vi "BinF_ReadData.vi"(6 "Channel number":i64, 7 "BinF File Settings":T1={"Version"=2, "Data Representation"=enum."I16", "# columns (samples per channel)"=300, "# rows (channels)"=150, "# pre-trigger samples"=20, "Sample rate"=1000.0, "ADC offset"=256.0, "Scale factor"=0.001}, 8 "error in":errorcluster, 9 "Length":i32, 10 "Start":i64, 11 "refnum":refnum<file>) -> (0 "error out":errorcluster, 1 "Unscaled data":sgl[](array[numeric]), 2 "Channel Data":sgl[](array[numeric]), 3 "refnum out":refnum<file>)   [LabVIEW 2021]
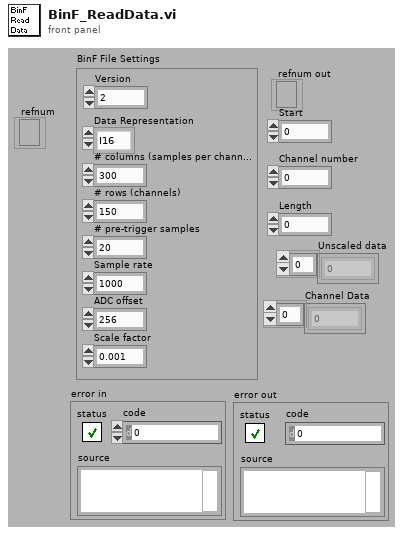
[diagram p1: front panel]
types:
  T1 = cluster{"Version":i16, "Data Representation":enum16{"Undefined", "I8", "I16", "I32", "I64", "U8", "U16", "U32", "U64", "SGL", "DBL", "EXT"}, "# columns (samples per channel)":i64, "# rows (channels)":i64, "# pre-trigger samples":i64, "Sample rate":dbl, "ADC offset":dbl, "Scale factor":dbl}
  T2 = enum16{"Undefined", "I8", "I16", "I32", "I64", "U8", "U16", "U32", "U64", "SGL", "DBL", "EXT"}
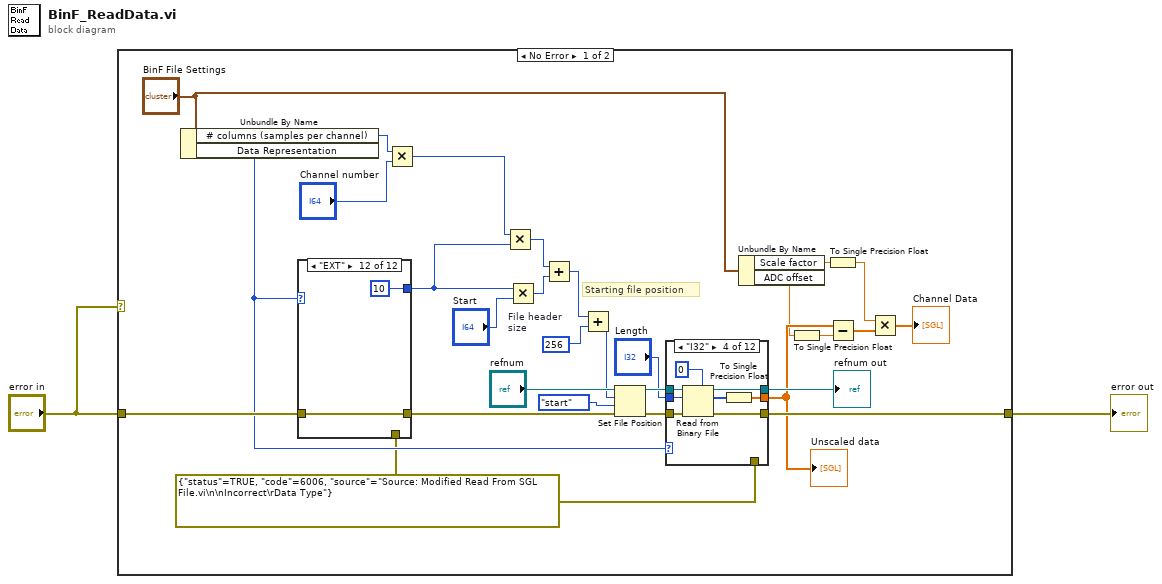
[diagram p0: block diagram]
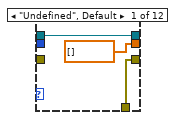
[diagram p2: hidden frame]
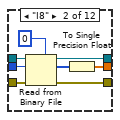
[diagram p3: hidden frame]
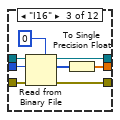
[diagram p4: hidden frame]
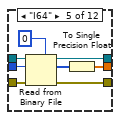
[diagram p5: hidden frame]
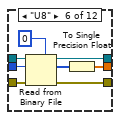
[diagram p6: hidden frame]
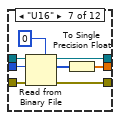
[diagram p7: hidden frame]
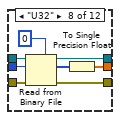
[diagram p8: hidden frame]
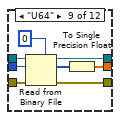
[diagram p9: hidden frame]
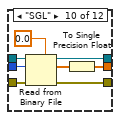
[diagram p10: hidden frame]
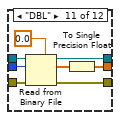
[diagram p11: hidden frame]
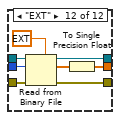
[diagram p12: hidden frame]
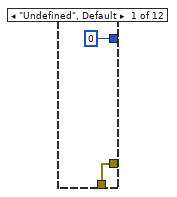
[diagram p13: hidden frame]
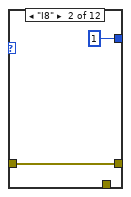
[diagram p14: hidden frame]
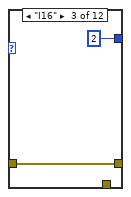
[diagram p15: hidden frame]
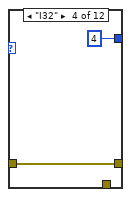
[diagram p16: hidden frame]
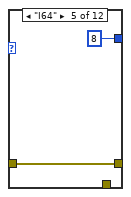
[diagram p17: hidden frame]
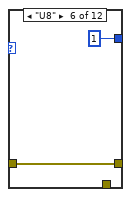
[diagram p18: hidden frame]
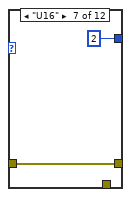
[diagram p19: hidden frame]
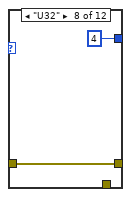
[diagram p20: hidden frame]
diagram:
  n1 = case shown="No Error" "error in" {
    tunnel: [w22 w147] -> w2
    tunnel: "error in" -> [w11 w147]
    frame No Error {
      w5 = errorcluster {"status"=TRUE, "code"=6006, "source"="Source: Modified Read From SGL File.vi\n\nIncorrect\rData Type"} ("error out")
      w7 = i64 256  # File header size
      # "Starting file position"
      n2 = Unbundle By Name("BinF File Settings") -> ("# columns (samples per channel)"=w25:i64, "Data Representation"=w6:T2)
      n3 = case shown="\"EXT\"" w6 {
        tunnel: [w124 w126 w128 w130 w132 w134 w136 w138 w140 w142 w144 w146] -> w13
        tunnel: w5 -> [w124 _ _ _ _ _ _ _ _ _ _ _]
        tunnel: [i64 0 i64 1 i64 2 i64 4 i64 8 i64 1 i64 2 i64 4 i64 8 i64 4 i64 8 i64 10] -> w12
        tunnel: w11 -> [_ w126 w128 w130 w132 w134 w136 w138 w140 w142 w144 w146]
        frame "Undefined", Default {
        }
        frame "I8" {
        }
        frame "I16" {
        }
        frame "I32" {
        }
        frame "I64" {
        }
        frame "U8" {
        }
        frame "U16" {
        }
        frame "U32" {
        }
        frame "U64" {
        }
        frame "SGL" {
        }
        frame "DBL" {
        }
        frame "EXT" {
        }
      }
      n4 = Multiply(x=w25, y="Channel number") -> (x*y=w19:i64)
      n5 = Multiply(x=w19, y=w12) -> (x*y=w10:i64)
      n6 = Multiply(x=w12, y="Start") -> (x*y=w9:i64)
      n7 = Add(x=w10, y=w9) -> (x+y=w8:i64)
      n8 = Add(x=w8, y=w7) -> (x+y=w26:i64)
      n9 = Set File Position(offset (in bytes) (0)=w26, refnum="refnum", from (0:start)=enum16{"start", "end", "current"}."start", error in=w13) -> (refnum out=w28:refnum<file>, error out=w29:errorcluster)
      n10 = case shown="\"I32\"" w6 {
        tunnel: w29 -> [_ w42 w50 w58 w66 w74 w82 w90 w98 w106 w114 w122]
        tunnel: w28 -> [w33 w41 w49 w57 w65 w73 w81 w89 w97 w105 w113 w121]
        tunnel: "Length" -> [_ w40 w48 w56 w64 w72 w80 w88 w96 w104 w112 w120]
        tunnel: [w34 w39 w47 w55 w63 w71 w79 w87 w95 w103 w111 w119] -> w22
        tunnel: [w33 w38 w46 w54 w62 w70 w78 w86 w94 w102 w110 w118] -> w21
        tunnel: [sgl[] [] w36 w44 w52 w60 w68 w76 w84 w92 w100 w108 w116] -> w20
        tunnel: w5 -> [w34 _ _ _ _ _ _ _ _ _ _ _]
        frame "Undefined", Default {
        }
        frame "I8" {
          n11 = Read from Binary File(5:i8 0, 8:w42, 10:w40, 11:w41) -> (0:w39:errorcluster, 2:w37:i8[], 3:w38:refnum<file>)  [unwired: 3 out]
          n12 = To Single Precision Float(number=w37) -> (single precision float=w36:sgl[])
        }
        frame "I16" {
          n13 = Read from Binary File(5:i16 0, 8:w50, 10:w48, 11:w49) -> (0:w47:errorcluster, 2:w45:i16[], 3:w46:refnum<file>)  [unwired: 3 out]
          n14 = To Single Precision Float(number=w45) -> (single precision float=w44:sgl[])
        }
        frame "I32" {
          n15 = Read from Binary File(5:0, 8:w58, 10:w56, 11:w57) -> (0:w55:errorcluster, 2:w53:i32[], 3:w54:refnum<file>)  [unwired: 3 out]
          n16 = To Single Precision Float(number=w53) -> (single precision float=w52:sgl[])
        }
        frame "I64" {
          n17 = Read from Binary File(5:i64 0, 8:w66, 10:w64, 11:w65) -> (0:w63:errorcluster, 2:w61:i64[], 3:w62:refnum<file>)  [unwired: 3 out]
          n18 = To Single Precision Float(number=w61) -> (single precision float=w60:sgl[])
        }
        frame "U8" {
          n19 = Read from Binary File(5:u8 0, 8:w74, 10:w72, 11:w73) -> (0:w71:errorcluster, 2:w69:u8[], 3:w70:refnum<file>)  [unwired: 3 out]
          n20 = To Single Precision Float(number=w69) -> (single precision float=w68:sgl[])
        }
        frame "U16" {
          n21 = Read from Binary File(5:u16 0, 8:w82, 10:w80, 11:w81) -> (0:w79:errorcluster, 2:w77:u16[], 3:w78:refnum<file>)  [unwired: 3 out]
          n22 = To Single Precision Float(number=w77) -> (single precision float=w76:sgl[])
        }
        frame "U32" {
          n23 = Read from Binary File(5:u32 0, 8:w90, 10:w88, 11:w89) -> (0:w87:errorcluster, 2:w85:u32[], 3:w86:refnum<file>)  [unwired: 3 out]
          n24 = To Single Precision Float(number=w85) -> (single precision float=w84:sgl[])
        }
        frame "U64" {
          n25 = Read from Binary File(5:u64 0, 8:w98, 10:w96, 11:w97) -> (0:w95:errorcluster, 2:w93:u64[], 3:w94:refnum<file>)  [unwired: 3 out]
          n26 = To Single Precision Float(number=w93) -> (single precision float=w92:sgl[])
        }
        frame "SGL" {
          n27 = Read from Binary File(5:sgl 0.0, 8:w106, 10:w104, 11:w105) -> (0:w103:errorcluster, 2:w101:sgl[], 3:w102:refnum<file>)  [unwired: 3 out]
          n28 = To Single Precision Float(number=w101) -> (single precision float=w100:sgl[])
        }
        frame "DBL" {
          n29 = Read from Binary File(5:0.0, 8:w114, 10:w112, 11:w113) -> (0:w111:errorcluster, 2:w109:dbl[], 3:w110:refnum<file>)  [unwired: 3 out]
          n30 = To Single Precision Float(number=w109) -> (single precision float=w108:sgl[])
        }
        frame "EXT" {
          n31 = Read from Binary File(5:ext 0.0, 8:w122, 10:w120, 11:w121) -> (0:w119:errorcluster, 2:w117:ext[], 3:w118:refnum<file>)  [unwired: 3 out]
          n32 = To Single Precision Float(number=w117) -> (single precision float=w116:sgl[])
        }
      }
      "refnum out" <- w21
      "Unscaled data" <- w20
      n33 = Unbundle By Name("BinF File Settings") -> ("Scale factor"=w16:dbl, "ADC offset"=w14:dbl)
      n34 = To Single Precision Float(number=w14) -> (single precision float=w4:sgl)
      n35 = To Single Precision Float(number=w16) -> (single precision float=w3:sgl)
      n36 = Subtract(x=w20, y=w4) -> (x-y=w17:sgl[])
      n37 = Multiply(x=w3, y=w17) -> (x*y=→"Channel Data":sgl[])
    }
    frame Error {
    }
  }
  "error out" <- w2
